vi "Stop Core.vi"(10 "final error code":i32, 11 "SubPanel Grid View in":refnum<class "SubPanel Grid View.lvclass">) -> (3 "SubPanel Grid View out":refnum<class "SubPanel Grid View.lvclass">)   [LabVIEW 2012, in "Win8uiDemo.lvlib" / "SubPanel Grid View.lvclass"]
doc: "(<B>Filename</B>: Actor Framework.lvlib:Actor.lvclass:Stop Core.vi)\n\nDefines what the actor does before it stops. Use the <B>final error code</B> input to determine whether the actor shut down in response to an error.\n\nBy default, this method does nothing. A descendant class may override it to define behavior, such as shutting down any processes the actor initiated in its override of the Actor Core method."
uses:
  SubPanel Grid View.lvclass
  SubPanel Grid View.lvclass/SubPanel Grid View.ctl
  Win8uiFramework/MainView.lvclass
  <vilib>/ActorFramework/Message Enqueuer/Message Enqueuer.lvclass/Message Enqueuer.ctl
  Read ViewableActor Enqueuers.vi
  <vilib>/ActorFramework/Message Enqueuer/Enqueue.vi
  <vilib>/ActorFramework/Message Priority Queue/Priority Enqueue.vi
  <vilib>/ActorFramework/Stop Msg/Stop Msg.lvclass
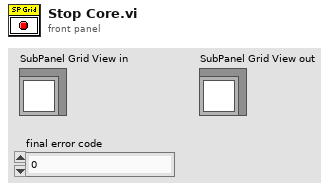
[diagram p1: front panel]
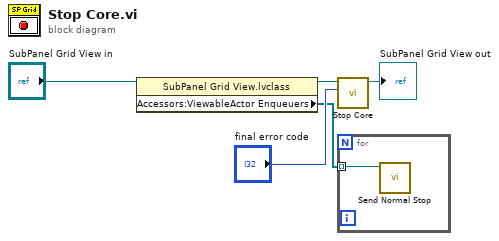
[diagram p0: block diagram]
diagram:
  n1 = property class="SubPanel Grid View.lvclass"(reference="SubPanel Grid View in") -> (reference out=w2:refnum<class "SubPanel Grid View.lvclass">, "Accessors:ViewableActor Enqueuers"=w1:refnum<class "Message Enqueuer.lvclass">[])  [unwired: 1 in, 1 out]
  n2 = call-parent "Stop Core.vi"("final error code"="final error code", "ViewableActor in"=w2) -> ("ViewableActor out"=→"SubPanel Grid View out":refnum<class "SubPanel Grid View.lvclass">)  [unwired: 9 in]
  n3 = for {
    tunnel: w1 -> [w6] mode=indexing
    n4 = call <vilib>:"Send Normal Stop.vi"("Message Enqueuer"=w6) -> ()  [unwired: 10 in, 1 out]
  }
